vi "MAX-Min.vi"() -> ()   [LabVIEW 2017]
panel:
  out "Array - Numeric":dbl[](array[numeric])
  out "min index":i32
  out "max index":i32
  out "min":dbl
  out "max":dbl
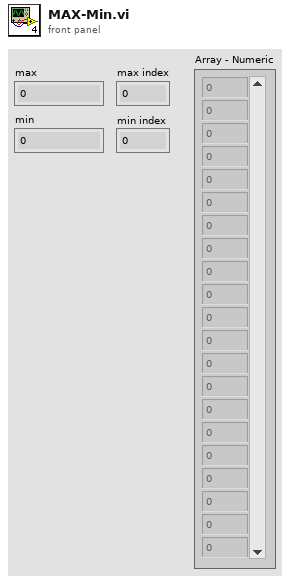
[diagram p1: front panel]
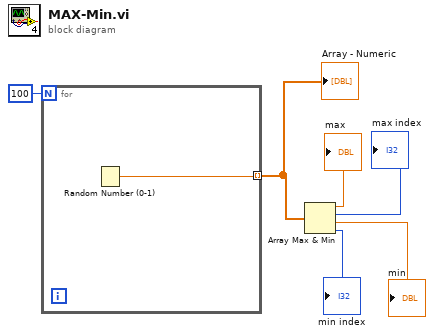
[diagram p0: block diagram]
diagram:
  n1 = for {
    N: 100 -> [_]
    tunnel: [w7] -> w1 mode=indexing
    n2 = Random Number (0-1)() -> (number: 0 to 1=w7:dbl)
  }
  "Array - Numeric" <- w1
  n3 = Array Max & Min(array=w1) -> (max value=→"max":dbl, max index (indices)=→"max index":i32, min value=→"min":dbl, min index (indices)=→"min index":i32)
